vi "Initialize-status-notifiers.vi"(8 "error in (no error)":errorcluster, 11 "ModComm in":T1) -> (0 "error out":errorcluster, 3 "ModComm out":T1)   [LabVIEW 2013, in "SLMServer.lvlib" / "SLMServer.lvclass"]
uses:
  SLMServer.lvclass
  Object-reference.ctl
  SLMServer.lvclass/SLMServer.ctl
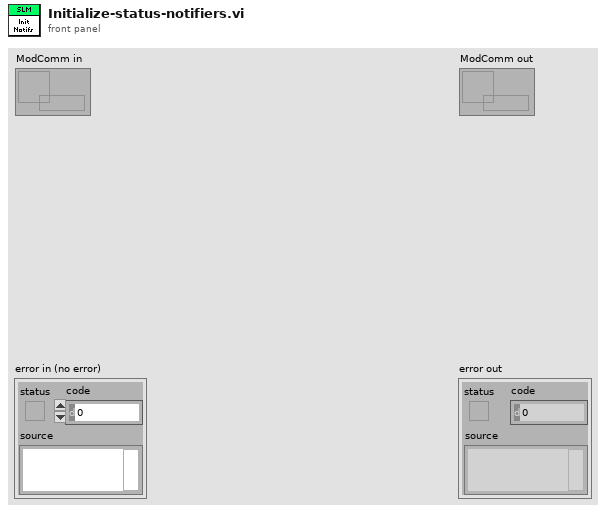
[diagram p1: front panel]
types:
  T1 = typedef "SLMServer.lvlib/SLMServer.lvclass/Object-reference.ctl" = refnum<data-value>
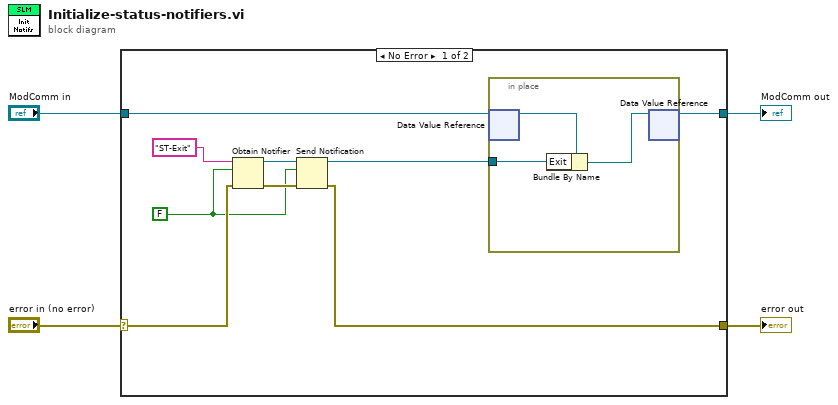
[diagram p0: block diagram]
diagram:
  n1 = case shown="No Error" "error in (no error)" {
    selector: "error in (no error)" -> [w12 w18]
    tunnel: [w8 w18] -> w3
    tunnel: [w10 w17] -> w1
    tunnel: "ModComm in" -> [w11 w17]
    frame No Error {
      w7 = FALSE
      n2 = Obtain Notifier(name (unnamed)="ST-Exit", notification data type=w7, error in (no error)=w12) -> (notifier out=w6:refnum<notifier>, error out=w9:errorcluster)  [unwired: 1 in, 1 out]
      n3 = Send Notification(notification=w7, notifier=w6, error in (no error)=w9) -> (notifier out=w5:refnum<notifier>, error out=w8:errorcluster)
      n4 = in-place {
        in-place-border: w5 -> [w16]
        n5 = in-place-dvr #1(w11) -> (w15:refnum<class "SLMServer.lvclass">)  [unwired: 1 out]
        n6 = Bundle By Name(cluster=w15, "Exit"=w16) -> (w14:refnum<class "SLMServer.lvclass">)
        n7 = in-place-dvr #1(w14) -> (w10:T1)  [unwired: 1 out]
      }
    }
    frame Error {
    }
  }
  "error out" <- w3
  "ModComm out" <- w1
